vi "Read Configuration.vi"(8 "file path (trajectorymat)":path=path "c:/ni-rt/startup/trajectorymat.csv", 9 "file path (matrixmat)":path=path "c:/ni-rt/startup/matrixmat_tuned_QR_7.csv", 10 "XML File Path conf":path=path "c:/ni-rt/startup/configuration.xml", 11 "Error In":errorcluster) -> (0 "values loded in xml files":T2, 1 "configuration":T1={"Accelerometer Bias"={"X (m/s)"=0.0, "Y (m/s)"=0.0, "Z (m/s)"=0.0}, "Gyroscope Bias"={"X (m/s)"=0.0, "Y (m/s)"=0.0, "Z (m/s)"=0.0}, "Steering Motor Gear Ratio"=111.0, "Steering Pully Gear Ratio"=1.0, "Steering Encoder CPR"=500.0, "Steering Motor Max RPM"=4000.0, "Wheelbase (m)"=1.12, "Fork Angle (rad)"=1.3, "Balancing Controller"={"Kp (/s)"=1.3, "Kd (1)"=3.0}, "Max Allowed Steering Angle (rad)"=0.7, "Task Periods"={"Emergency Stop (us)"=10000, "IMU (us)"=10000, "Steering Motor Encoder (us)"=10000, "State Estimator (us)"=10000, "Balancing Controller (us)"=10000, "GNSS (us)"=10000, "Logging (us)"=50000, "Drive Motor (us)"=100000, "Visualization (us)"=100000}, "Drive Motor Gear Ratio"=250.0, "lr"=0.4964, "lf"=0.5986, "lambda"=1.2217, "k1"=0.004472, "k2"=0.09678, "e1_max"=11.331, "Ad_tmin"=0.95971, "Bd_tmin"=0.01, "C_tmin"=2.20588, "D_tmin"=0.0, "Wheel radius"=0.311, "Ad_tmax"=0.95971, "Bd_tmax"=0.01, "C_tmax"=2.20588, "D_tmax"=0.0, "Vmin"=2.20588, "Vmax"=0.0}, 2 "value":T3, 3 "error out":errorcluster, 4 "Trajectory":T3, 5 "Init trajectory (2)":dbl[][](array[numeric]), 6 "Matrix Matlab":T3)   [LabVIEW 2021]
uses:
  <vilib>/Analysis/Matrix/Datatypes/RealMatrix.ctl
  Configuration.ctl
  <vilib>/Utility/xml.llb/Read From XML File(string).vi
  <vilib>/Analysis/Matrix/Numeric/Conversions/Matrix To Array - RM.vi
  <vilib>/Utility/file.llb/Read Delimited Spreadsheet (DBL).vi
  <vilib>/Analysis/Matrix/NI_Matrix.lvlib
panel:
  in  "delimiter (,) 2":string=","
  in  "error in (no error) 2":errorcluster
  in  "delimiter (,)":string=","
  in  "error in (no error)":errorcluster
  in  "init trajectory":dbl[][](array[numeric])
  in  "XML File Path traj":path=path "c:/ni-rt/startup/trajectorylab.xml"
  in  "Init Matrix":T3
  in  "XML File Path matr":path=path "c:/ni-rt/startup/matrixlab.xml"
  # "e"
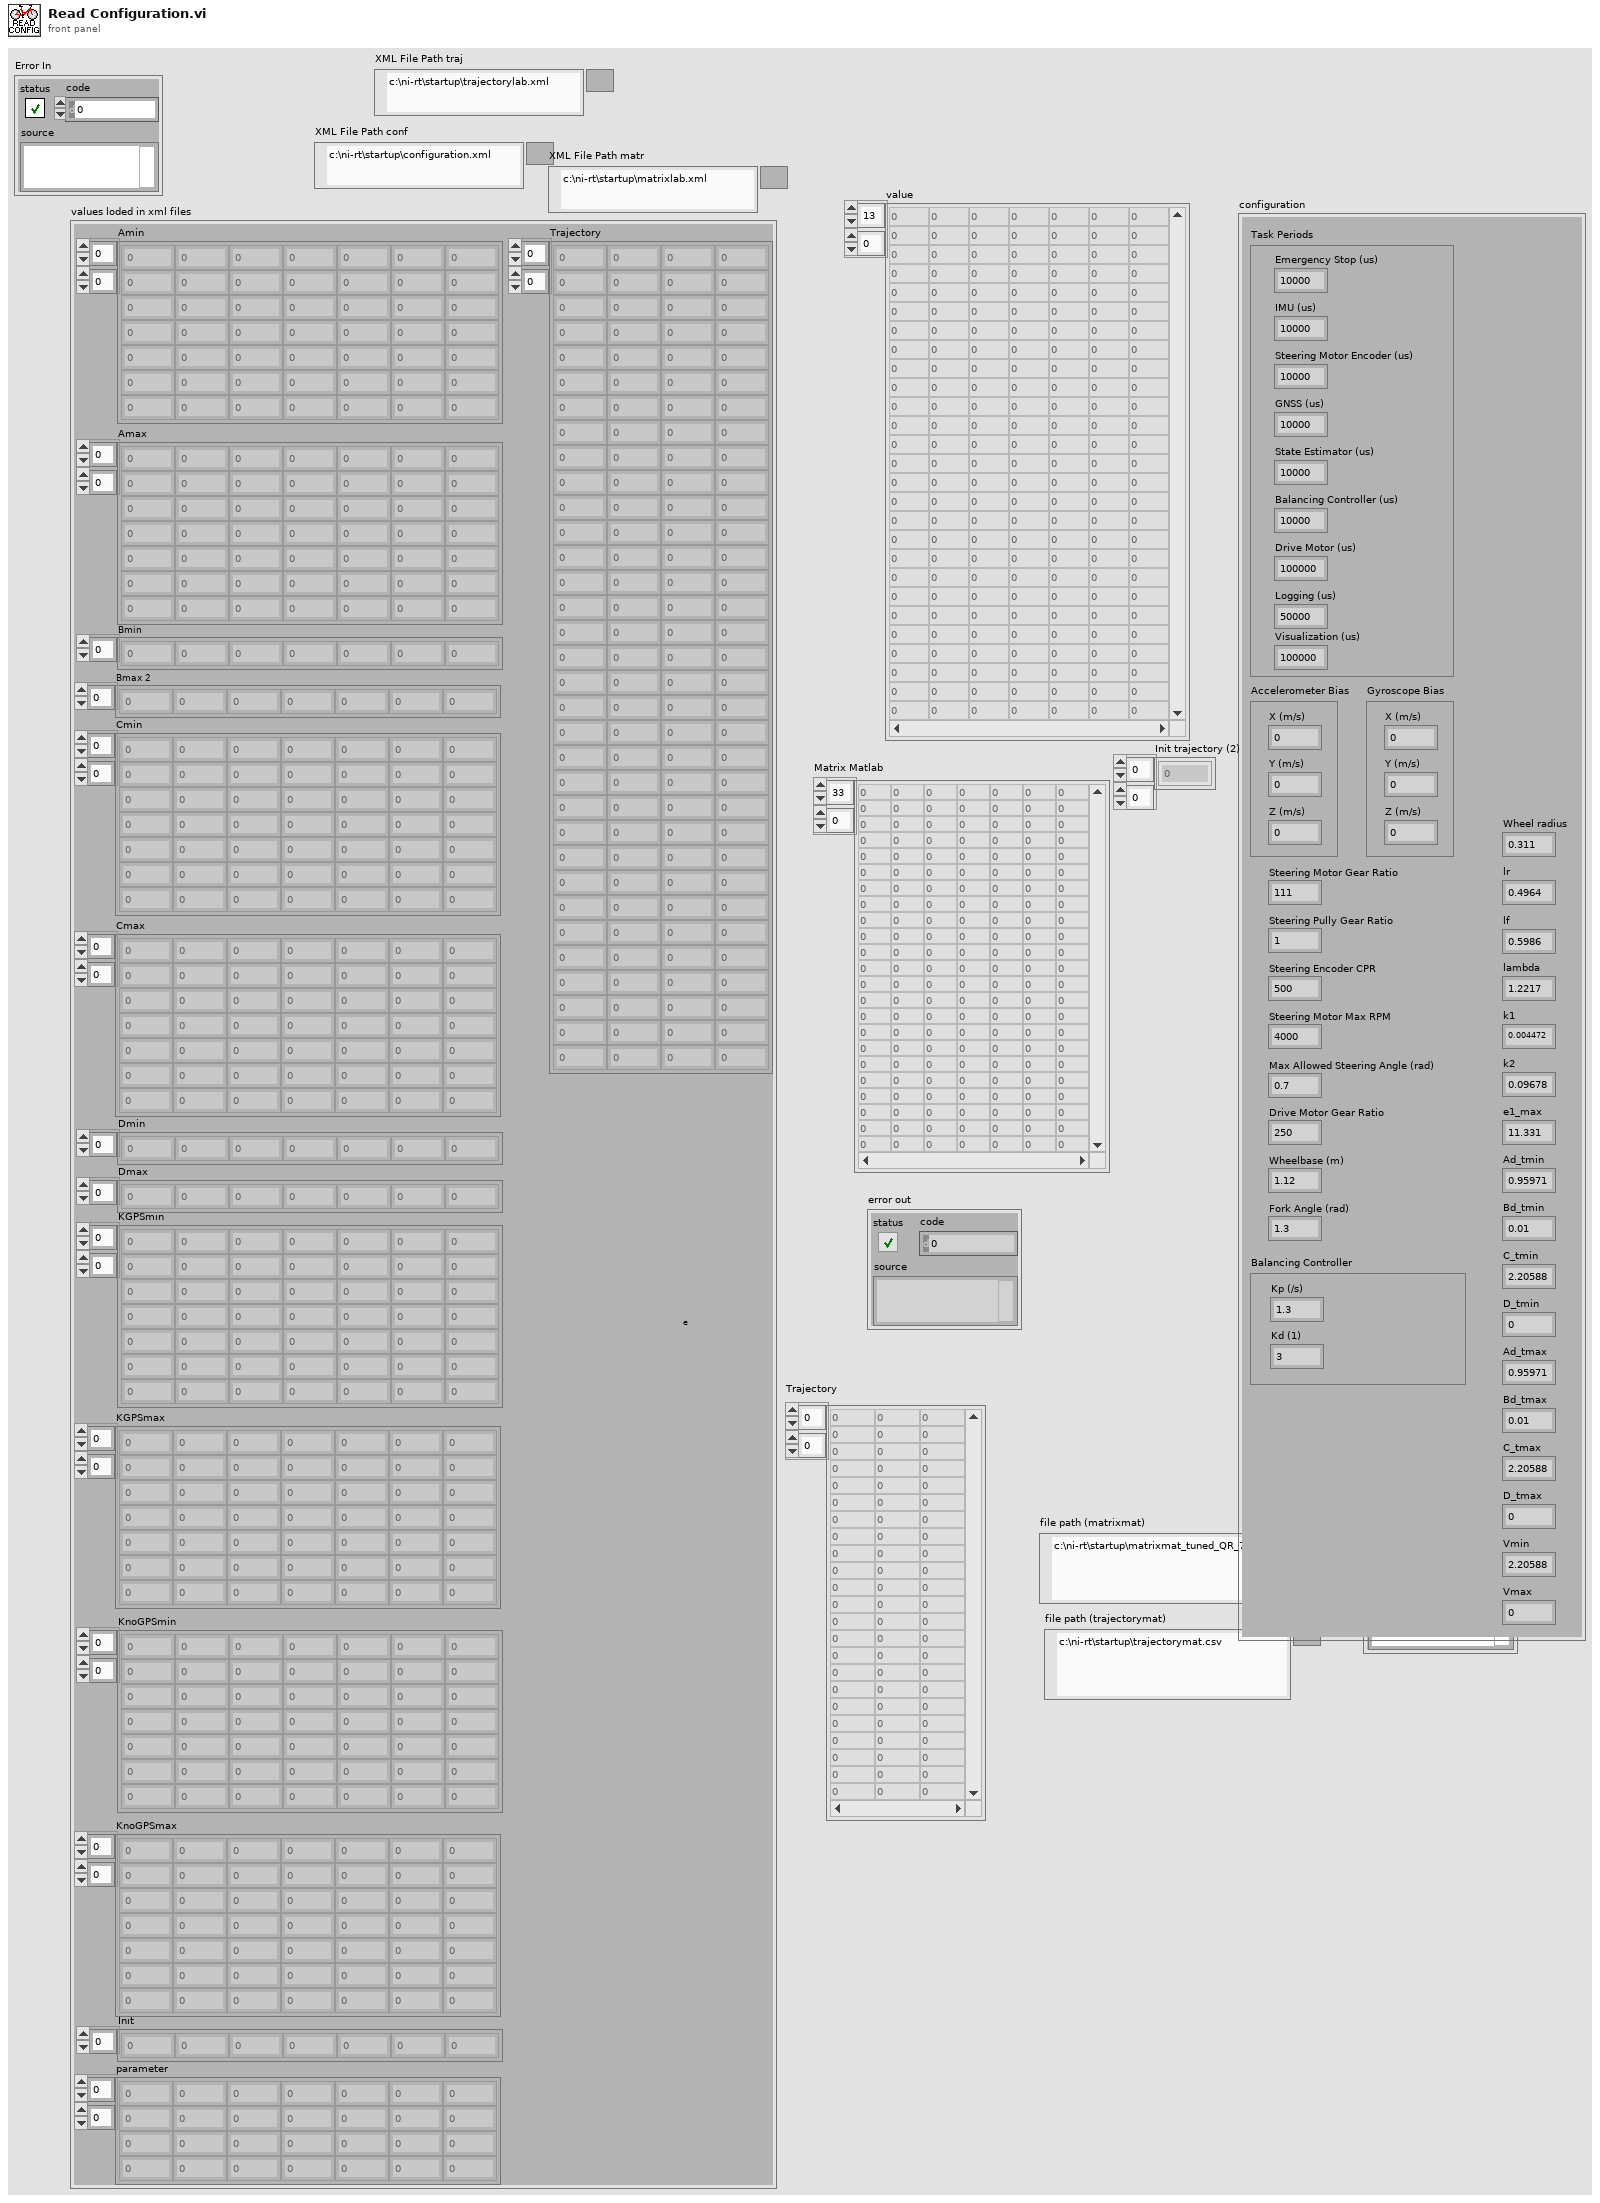
[diagram p1: front panel]
types:
  T1 = typedef "Configuration.ctl" = cluster{"Accelerometer Bias":cluster{"X (m/s)":dbl, "Y (m/s)":dbl, "Z (m/s)":dbl}, "Gyroscope Bias":cluster{"X (m/s)":dbl, "Y (m/s)":dbl, "Z (m/s)":dbl}, "Steering Motor Gear Ratio":dbl, "Steering Pully Gear Ratio":dbl, "Steering Encoder CPR":dbl, "Steering Motor Max RPM":dbl, "Wheelbase (m)":dbl, "Fork Angle (rad)":dbl, "Balancing Controller":cluster{"Kp (/s)":dbl, "Kd (1)":dbl}, "Max Allowed Steering Angle (rad)":dbl, "Task Periods":cluster{"Emergency Stop (us)":i64, "IMU (us)":i64, "Steering Motor Encoder (us)":i64, "State Estimator (us)":i64, "Balancing Controller (us)":i64, "GNSS (us)":i64, "Logging (us)":i64, "Drive Motor (us)":i64, "Visualization (us)":i64}, "Drive Motor Gear Ratio":dbl, "lr":dbl, "lf":dbl, "lambda":dbl, "k1":dbl, "k2":dbl, "e1_max":dbl, "Ad_tmin":dbl, "Bd_tmin":dbl, "C_tmin":dbl, "D_tmin":dbl, "Wheel radius":dbl, "Ad_tmax":dbl, "Bd_tmax":dbl, "C_tmax":dbl, "D_tmax":dbl, "Vmin":dbl, "Vmax":dbl}
  T2 = cluster{"Bmin":dbl[], "Amin":dbl[][], "Cmin":dbl[][], "Dmin":dbl[], "KGPSmin":dbl[][], "Trajectory":dbl[][], "Init":dbl[], "parameter":dbl[][], "KnoGPSmin":dbl[][], "Amax":dbl[][], "Bmax 2":dbl[], "Cmax":dbl[][], "Dmax":dbl[], "KGPSmax":dbl[][], "KnoGPSmax":dbl[][]}
  T3 = typedef "NI_Matrix.lvlib/RealMatrix.ctl" = dbl[][]
  T4 = cluster{"Bmin":dbl[], "Amin":dbl[][], "Cmin":dbl[][], "Dmin":dbl[], "KGPSmin":dbl[][], "Trajectory":dbl[][], "Init":dbl[], "parameter":dbl[][], "KnoGPSmin":dbl[][], "Amax":dbl[][], "Bmax":dbl[], "Cmax":dbl[][], "Dmax":dbl[], "KGPSmax":dbl[][], "KnoGPSmax":dbl[][]}
  T5 = cluster{"[0]":dbl, "[1]":dbl, "[2]":dbl, "[3]":dbl, "[4]":dbl, "[5]":dbl, "[6]":dbl, "[7]":dbl, "[8]":dbl, "[9]":dbl, "[10]":dbl, "[11]":dbl, "[12]":dbl, "[13]":dbl, "[14]":dbl, "[15]":dbl, "[16]":dbl, "[17]":dbl, "[18]":dbl, "[19]":dbl, "[20]":dbl, "[21]":dbl, "[22]":dbl, "[23]":dbl, "[24]":dbl, "[25]":dbl, "[26]":dbl, "[27]":dbl}
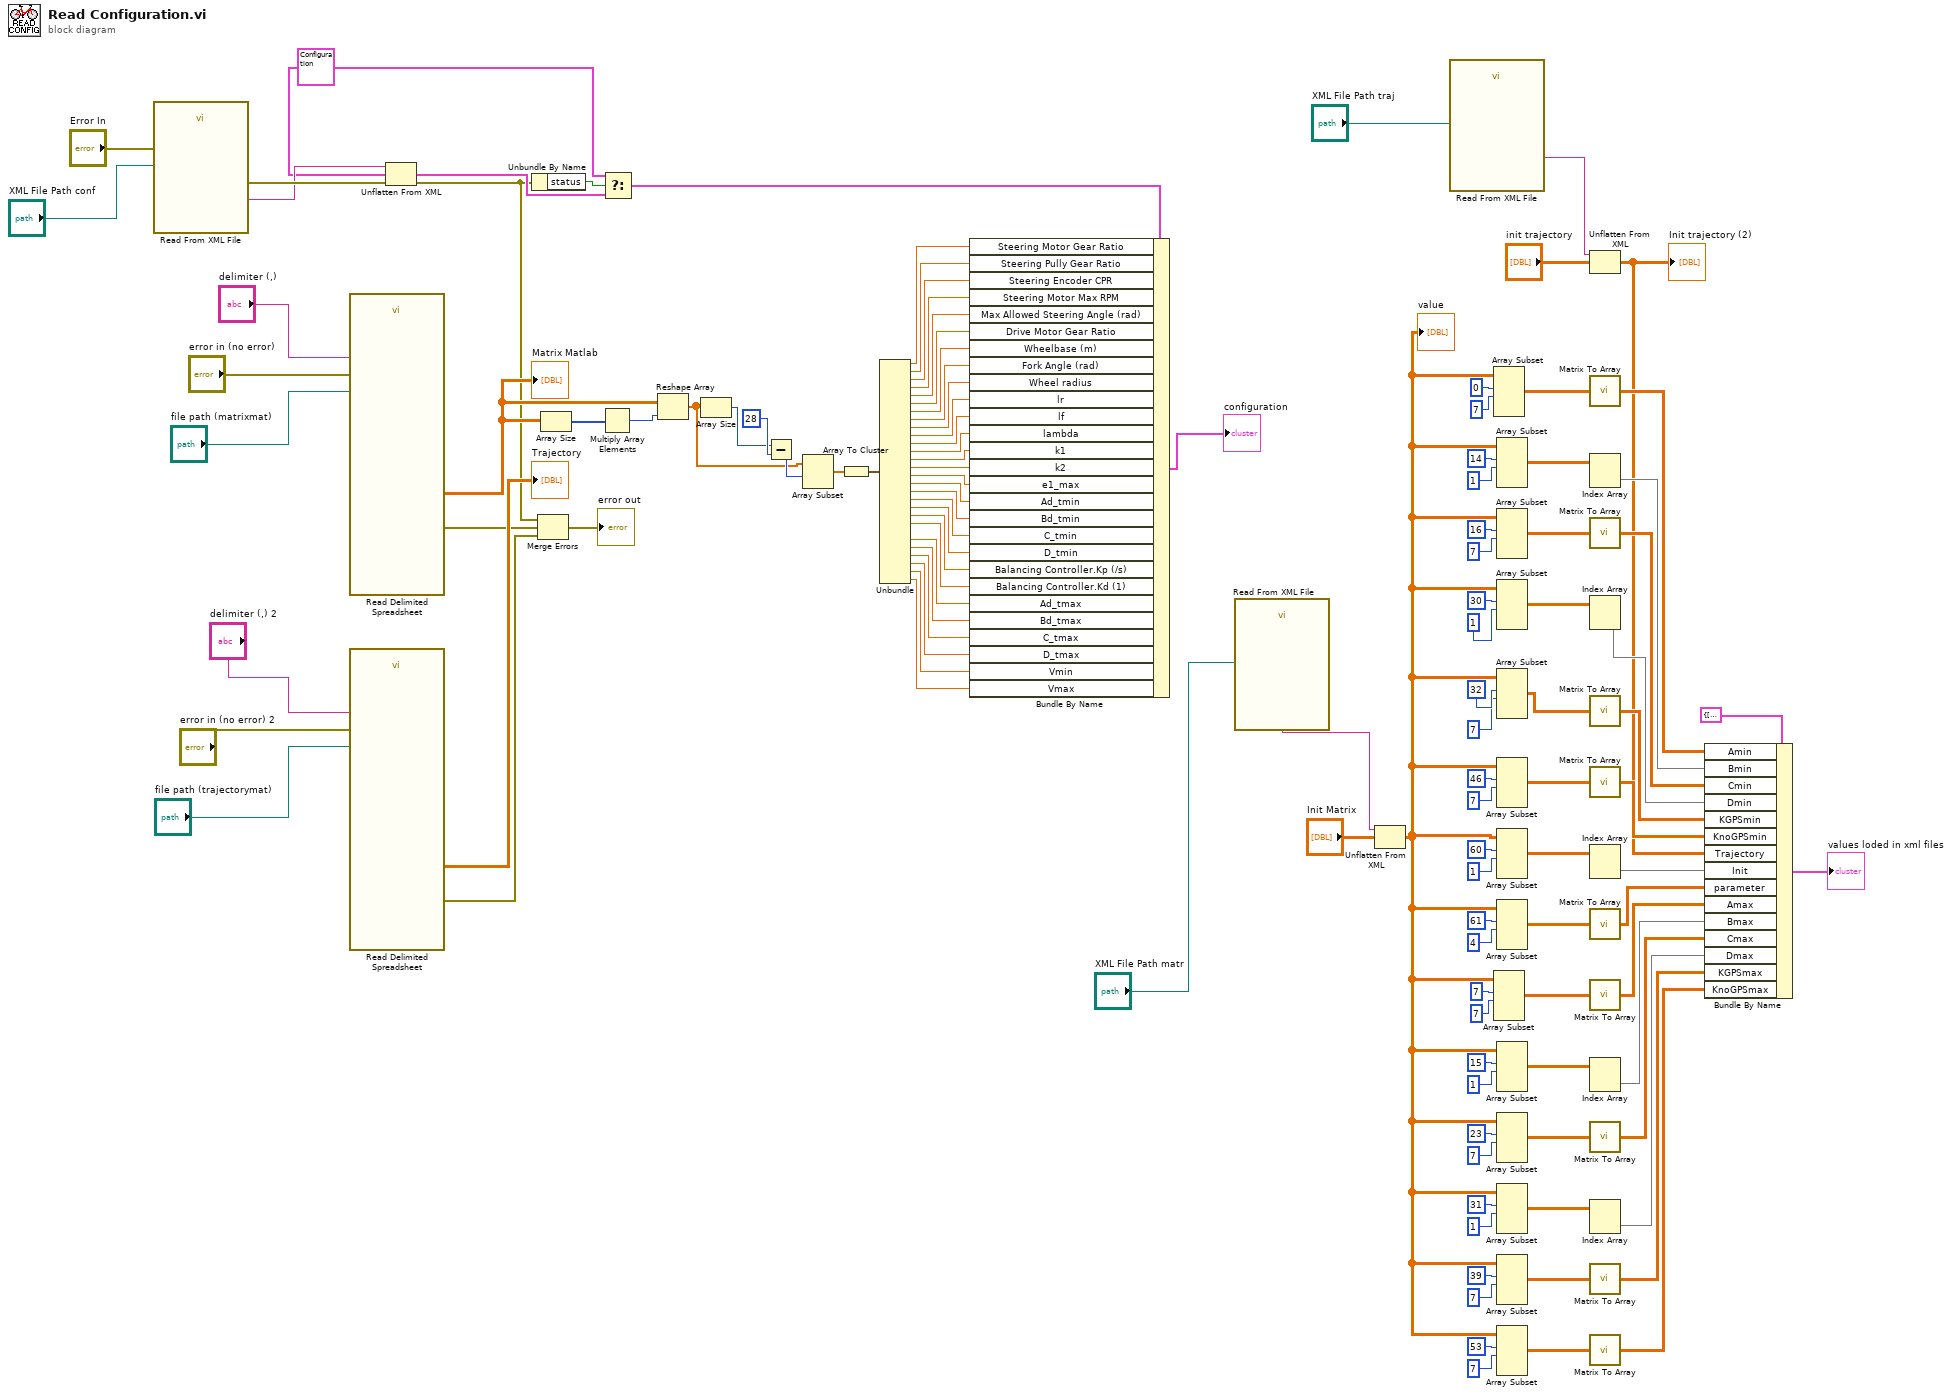
[diagram p0: block diagram]
diagram:
  w58 = T1 {"Accelerometer Bias"={"X (m/s)"=0.0, "Y (m/s)"=0.0, "Z (m/s)"=0.0}, "Gyroscope Bias"={"X (m/s)"=0.0, "Y (m/s)"=0.0, "Z (m/s)"=0.0}, "Steering Motor Gear Ratio"=611.0, "Steering Pully Gear Ratio"=1.0, "Steering Encoder CPR"=500.0, "Steering Motor Max RPM"=4000.0, "Wheelbase (m)"=1.12, "Fork Angle (rad)"=1.3, "Balancing Controller"={"Kp (/s)"=0.0, "Kd (1)"=0.0}, "Max Allowed Steering Angle (rad)"=0.7, "Task Periods"={"Emergency Stop (us)"=0, "IMU (us)"=0, "Steering Motor Encoder (us)"=0, "State Estimator (us)"=0, "Balancing Controller (us)"=0, "GNSS (us)"=0, "Logging (us)"=0, "Drive Motor (us)"=0, "Visualization (us)"=50000}, "Drive Motor Gear Ratio"=0.7, "lr"=0.0, "lf"=0.0, "lambda"=0.0, "k1"=0.0, "k2"=0.0, "e1_max"=0.0, "Ad_tmin"=0.0, "Bd_tmin"=0.0, "C_tmin"=0.0, "D_tmin"=0.0, "Wheel radius"=0.311, "Ad_tmax"=0.95971, "Bd_tmax"=0.01, "C_tmax"=2.20588, "D_tmax"=0.0, "Vmin"=2.20588, "Vmax"=0.0} ("Configuration")
  n1 = call-poly <vilib>:"Read From XML File.vi"("error in (no error)"="Error In", "XML File Path"="XML File Path conf") -> ("error out"=w122:errorcluster, "XML Elements"=w121:string)  [unwired: 7 in, 1 out]
  n2 = call-poly <vilib>:"Read Delimited Spreadsheet.vi"("file path (dialog if empty)"="file path (matrixmat)", "error in (no error)"="error in (no error)", "delimiter (\\t)"="delimiter (,)") -> ("all rows"=w82:dbl[][], "error out"=w53:errorcluster)  [unwired: 7 in, 4 out]
  "Matrix Matlab" <- w82
  n3 = call-poly <vilib>:"Read Delimited Spreadsheet.vi"("file path (dialog if empty)"="file path (trajectorymat)", "error in (no error)"="error in (no error) 2", "delimiter (\\t)"="delimiter (,) 2") -> ("all rows"=→"Trajectory":dbl[][], "error out"=w52:errorcluster)  [unwired: 7 in, 4 out]
  n4 = Unflatten From XML(xml string=w121, type=w58, error in (no error)=w122) -> (value=w118:T1, error out=w54:errorcluster)
  n5 = Unbundle By Name(w54) -> ("status"=w115:bool)
  n6 = Merge Errors(w54, w53, w52) -> (→"error out":errorcluster)
  n7 = Array Size(array=w82) -> (size(s)=w87:i32[])
  n8 = Multiply Array Elements(1:w87) -> (0:w86:i32)
  n9 = Select(t=w58, s=w115, f=w118) -> (s? t:f=w57:T1)
  n10 = Reshape Array(w82, w86) -> (w81:dbl[])
  n11 = Array Size(array=w81) -> (size(s)=w84:i32)
  n12 = Subtract(x=w84, y=28 ("length")) -> (x-y=w83:i32)
  n13 = Array Subset(array=w81, index=w83) -> (w80:dbl[])  [unwired: 1 in]
  n14 = Array To Cluster(array=w80) -> (cluster=w79:T5)
  n15 = Unbundle(w79) -> ("[0]"=w78:dbl, "[1]"=w77:dbl, "[2]"=w76:dbl, "[3]"=w75:dbl, "[4]"=w74:dbl, "[5]"=w73:dbl, "[6]"=w72:dbl, "[7]"=w71:dbl, "[8]"=w70:dbl, "[9]"=w69:dbl, "[10]"=w68:dbl, "[11]"=w67:dbl, "[12]"=w66:dbl, "[13]"=w65:dbl, "[14]"=w64:dbl, "[15]"=w63:dbl, "[16]"=w62:dbl, "[17]"=w61:dbl, "[18]"=w60:dbl, "[19]"=w51:dbl, "[20]"=w59:dbl, "[22]"=w6:dbl, "[23]"=w5:dbl, "[24]"=w4:dbl, "[25]"=w3:dbl, "[26]"=w2:dbl, "[27]"=w1:dbl)  [unwired: 1 out]
  n16 = Bundle By Name(cluster=w57, "Steering Motor Gear Ratio"=w78, "Steering Pully Gear Ratio"=w77, "Steering Encoder CPR"=w76, "Steering Motor Max RPM"=w75, "Max Allowed Steering Angle (rad)"=w74, "Drive Motor Gear Ratio"=w73, "Wheelbase (m)"=w72, "Fork Angle (rad)"=w71, "Wheel radius"=w70, "lr"=w69, "lf"=w68, "lambda"=w67, "k1"=w66, "k2"=w65, "e1_max"=w64, "Ad_tmin"=w63, "Bd_tmin"=w62, "C_tmin"=w61, "D_tmin"=w60, "Balancing Controller.Kp (/s)"=w51, "Balancing Controller.Kd (1)"=w59, "Ad_tmax"=w6, "Bd_tmax"=w5, "C_tmax"=w4, "D_tmax"=w3, "Vmin"=w2, "Vmax"=w1) -> (→"configuration":T1)
  n17 = call-poly <vilib>:"Read From XML File.vi"("XML File Path"="XML File Path matr") -> ("XML Elements"=w116:string)  [unwired: 8 in, 2 out]
  n18 = Unflatten From XML(xml string=w116, type="Init Matrix") -> (value=w12:T3)  [unwired: 1 in, 1 out]
  "value" <- w12
  n19 = call-poly <vilib>:"Read From XML File.vi"("XML File Path"="XML File Path traj") -> ("XML Elements"=w101:string)  [unwired: 8 in, 2 out]
  n20 = Array Subset(array=w12, index (row)=0, length (row)=7) -> (w112:T3)  [unwired: 2 in]
  n21 = Array Subset(array=w12, index (row)=7, length (row)=7) -> (w47:T3)  [unwired: 2 in]
  n22 = Array Subset(array=w12, index (row)=14, length (row)=1) -> (w45:T3)  [unwired: 2 in]
  n23 = Array Subset(array=w12, index (row)=16, length (row)=7) -> (w41:T3)  [unwired: 2 in]
  n24 = Array Subset(array=w12, index (row)=30, length (row)=1) -> (w37:T3)  [unwired: 2 in]
  n25 = Array Subset(array=w12, index (row)=32, length (row)=7) -> (w29:T3)  [unwired: 2 in]
  n26 = Array Subset(array=w12, index (row)=46, length (row)=7) -> (w23:T3)  [unwired: 2 in]
  n27 = Array Subset(array=w12, index (row)=60, length (row)=1) -> (w13:T3)  [unwired: 2 in]
  n28 = Array Subset(array=w12, index (row)=61, length (row)=4) -> (w9:T3)  [unwired: 2 in]
  n29 = Array Subset(array=w12, index (row)=15, length (row)=1) -> (w43:T3)  [unwired: 2 in]
  n30 = Array Subset(array=w12, index (row)=23, length (row)=7) -> (w39:T3)  [unwired: 2 in]
  n31 = Array Subset(array=w12, index (row)=31, length (row)=1) -> (w33:T3)  [unwired: 2 in]
  n32 = Array Subset(array=w12, index (row)=39, length (row)=7) -> (w26:T3)  [unwired: 2 in]
  n33 = Array Subset(array=w12, index (row)=53, length (row)=7) -> (w17:T3)  [unwired: 2 in]
  n34 = Unflatten From XML(xml string=w101, type="init trajectory") -> (value=w10:dbl[][])  [unwired: 1 in, 1 out]
  "Init trajectory (2)" <- w10
  n35 = call-poly <vilib>:"Matrix To Array.vi"("Real Matrix"=w112) -> ("Real 2D Array"=w111:dbl[][])
  n36 = Index Array(array=w45) -> (element=w44:dbl[])  [unwired: 2 in]
  n37 = call-poly <vilib>:"Matrix To Array.vi"("Real Matrix"=w41) -> ("Real 2D Array"=w40:dbl[][])
  n38 = Index Array(array=w37) -> (element=w36:dbl[])  [unwired: 2 in]
  n39 = call-poly <vilib>:"Matrix To Array.vi"("Real Matrix"=w29) -> ("Real 2D Array"=w20:dbl[][])
  n40 = call-poly <vilib>:"Matrix To Array.vi"("Real Matrix"=w23) -> ("Real 2D Array"=w18:dbl[][])
  n41 = Index Array(array=w13) -> (element=w11:dbl[])  [unwired: 2 in]
  n42 = call-poly <vilib>:"Matrix To Array.vi"("Real Matrix"=w9) -> ("Real 2D Array"=w8:dbl[][])
  n43 = call-poly <vilib>:"Matrix To Array.vi"("Real Matrix"=w47) -> ("Real 2D Array"=w46:dbl[][])
  n44 = Index Array(array=w43) -> (element=w42:dbl[])  [unwired: 2 in]
  n45 = call-poly <vilib>:"Matrix To Array.vi"("Real Matrix"=w39) -> ("Real 2D Array"=w38:dbl[][])
  n46 = Index Array(array=w33) -> (element=w32:dbl[])  [unwired: 2 in]
  n47 = call-poly <vilib>:"Matrix To Array.vi"("Real Matrix"=w26) -> ("Real 2D Array"=w19:dbl[][])
  n48 = call-poly <vilib>:"Matrix To Array.vi"("Real Matrix"=w17) -> ("Real 2D Array"=w16:dbl[][])
  n49 = Bundle By Name(cluster=T4 {"Bmin"=[], "Amin"=[], "Cmin"=[], "Dmin"=[], "KGPSmin"=[], "Trajectory"=[], "Init"=[], "parameter"=[], "KnoGPSmin"=[], "Amax"=[], "Bmax"=[], "Cmax"=[], "Dmax"=[], "KGPSmax"=[], "KnoGPSmax"=[]} ("Matrix 2"), "Amin"=w111, "Bmin"=w44, "Cmin"=w40, "Dmin"=w36, "KGPSmin"=w20, "KnoGPSmin"=w18, "Trajectory"=w10, "Init"=w11, "parameter"=w8, "Amax"=w46, "Bmax"=w42, "Cmax"=w38, "Dmax"=w32, "KGPSmax"=w19, "KnoGPSmax"=w16) -> (→"values loded in xml files":T4)
